vi "ryerror_history.vi"(6 "reset? (F)":bool, 8 "error in (no error)":errorcluster, 9 "return elements? (T)":bool=TRUE) -> (0 "error out":errorcluster, 1 "history":errorcluster[](array[cluster]))   [LabVIEW 2017]
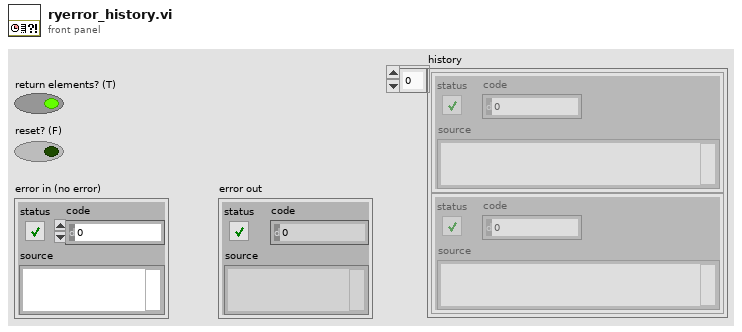
[diagram p1: front panel]
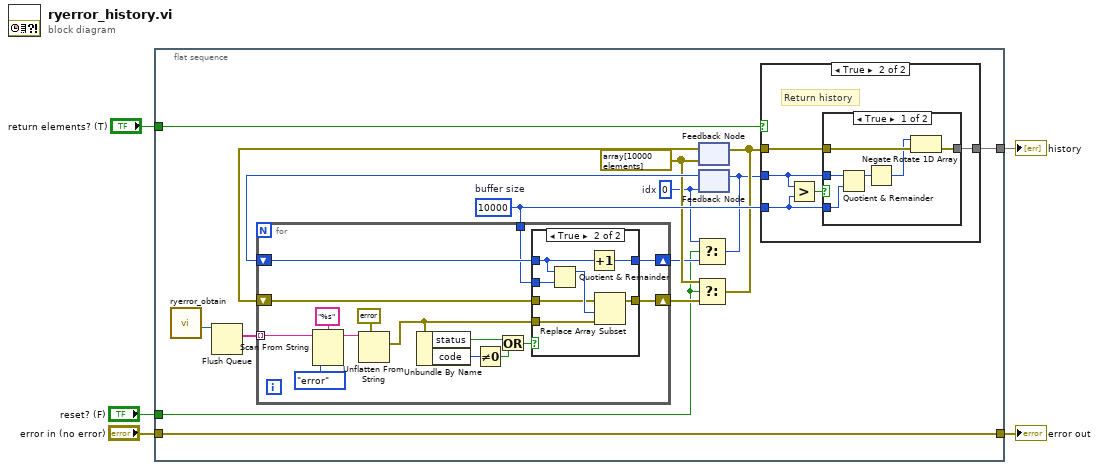
[diagram p0: block diagram]
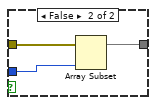
[diagram p4: hidden frame]
diagram:
  n1 = flat-sequence {
    tunnel: "reset? (F)" -> [w6]
    tunnel: [w17] -> w4
    tunnel: [w18] -> w3
    tunnel: "error in (no error)" -> [w18]
    tunnel: "return elements? (T)" -> [w15]
    frame #0 {
      w16 = 10000  # buffer size
      w7 = 0  # idx
      w10 = errorcluster[] array[10000 elements]
      n2 = call "ryerror_obtain.vi"() -> ("error queue"=w20:refnum<queue>)  [unwired: 10 in, 1 out]
      n3 = Flush Queue(queue=w20) -> (remaining elements=w19:string[])  [unwired: 1 in, 2 out]
      n4 = feedback #1(w10) -> (w13:errorcluster[])
      n5 = feedback #2(w7) -> (w14:i32)
      n6 = for {
        tunnel: w19 -> [w34] mode=indexing
        shift-right: [w26] -> w12
        shift-left: w13 -> [w27]
        shift-right: [w24] -> w9
        shift-left: w14 -> [w23]
        tunnel: w16 -> [w21]
        n7 = Scan From String(format string="%s", input string=w34, default 1=enum8{"error"}."error") -> (remaining string=w31:string)  [unwired: 3 in, 2 out]
        n8 = Unflatten From String(type=errorcluster {"status"=FALSE, "code"=0, "source"=""} ("error in (no error)"), binary string=w31) -> (value=w25:errorcluster)  [unwired: 3 in, 2 out]
        n9 = Unbundle By Name(w25) -> ("status"=w30:bool, "code"=w29:i32)
        n10 = Not Equal To 0?(x=w29) -> (x != 0?=w28:bool)
        n11 = Or(x=w30, y=w28) -> (x .or. y?=w22:bool)
        n12 = case shown="True" w22 {
          tunnel: w27 -> [w36 w39]
          tunnel: [w36 w44] -> w26
          tunnel: w25 -> [_ w43]
          tunnel: [w37 w42] -> w24
          tunnel: w23 -> [w37 w41]
          tunnel: w21 -> [_ w38]
          frame False {
          }
          frame True {
            n13 = Quotient & Remainder(x=w41, y=w38) -> (x-y*floor(x/y)=w40:i32)  [unwired: 1 out]
            n14 = Increment(x=w41) -> (x+1=w42:i32)
            n15 = Replace Array Subset(array=w39, new element=w43, index=w40) -> (w44:errorcluster[])
          }
        }
      }
      n16 = Select(t=w7, s=w6, f=w9) -> (s? t:f=w8:i32)
      n17 = Select(t=w10, s=w6, f=w12) -> (s? t:f=w11:errorcluster[])
      n18 = feedback-in #1(w11) -> ()
      n19 = feedback-in #2(w8) -> ()
      n20 = case shown="True" w15 {
        tunnel: w11 -> [_ w49]
        tunnel: [_ w48] -> w17
        tunnel: w8 -> [_ w46]
        tunnel: w16 -> [_ w45]
        frame False {
          # "Don't return history"
        }
        frame True {
          # "Return history"
          n21 = Greater?(x=w46, y=w45) -> (0:w47:bool)
          n22 = case shown="True" w47 {
            tunnel: w49 -> [w53 w58]
            tunnel: [w52 w57] -> w48
            tunnel: w46 -> [w55 w56]
            tunnel: w45 -> [w54 _]
            frame True {
              n23 = Quotient & Remainder(x=w55, y=w54) -> (x-y*floor(x/y)=w51:i32)  [unwired: 1 out]
              n24 = Negate(x=w51) -> (-x=w50:i32)
              n25 = Rotate 1D Array(1:w53, 2:w50) -> (0:w52:errorcluster[])
            }
            frame False {
              n26 = Array Subset(array=w58, length=w56) -> (w57:errorcluster[])  [unwired: 1 in]
            }
          }
        }
      }
    }
  }
  "error out" <- w3
  "history" <- w4
